vi "cargarDatoEstadistica.vi"(11 "IndiceAUltimoValor\nAgregadoEnLaTabla":i32=1) -> ()   [LabVIEW 2014]
uses:
  claseEstadistica/claseEstadistica.lvclass
panel:
  out "dataReading":T1
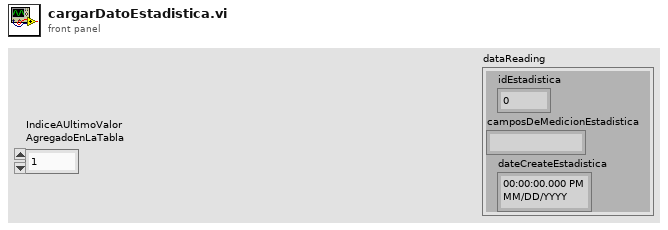
[diagram p1: front panel]
types:
  T1 = cluster{"idEstadistica":dbl, "camposDeMedicionEstadistica":string, "dateCreateEstadistica":timestamp}
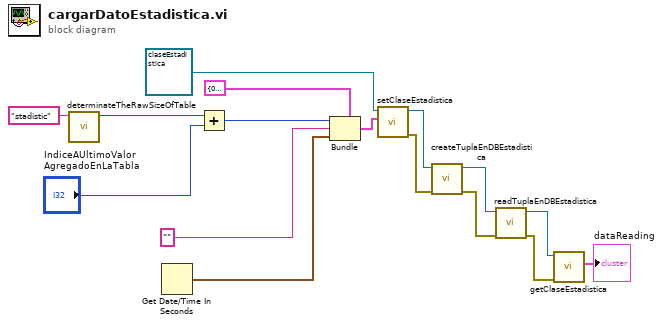
[diagram p0: block diagram]
diagram:
  n1 = call "determinateTheRawSizeOfTable.vi"("tableName"="stadistic") -> ("sizeOfTableInNumberRaw"=w3:i32)  [unwired: 8 in, 1 out]
  n2 = Get Date/Time In Seconds() -> (seconds since 1Jan1904=w14:timestamp)
  n3 = Add(x=w3, y="IndiceAUltimoValor\nAgregadoEnLaTabla") -> (x+y=w15:i32)
  n4 = Bundle(cluster=T1 {"idEstadistica"=0.0, "camposDeMedicionEstadistica"="", "dateCreateEstadistica"=timestamp(0 s since 1904-01-01)} ("dataToSet"), "idEstadistica"=w15, "camposDeMedicionEstadistica"="", "dateCreateEstadistica"=w14) -> (w10:T1)
  n5 = call "setClaseEstadistica.vi"("dataToSet"=w10, "claseEstadistica in"=refnum<class "claseEstadistica.lvclass"> refnum ("claseEstadistica.lvclass")) -> ("error out"=w8:errorcluster, "claseEstadistica out"=w9:refnum<class "claseEstadistica.lvclass">)  [unwired: 8 in]
  n6 = call "createTuplaEnDBEstadistica.vi"("error in"=w8, "claseEstadistica in"=w9) -> ("error out"=w6:errorcluster, "claseEstadistica out"=w7:refnum<class "claseEstadistica.lvclass">)  [unwired: 8 in]
  n7 = call "readTuplaEnDBEstadistica.vi"("error in"=w6, "claseEstadistica in"=w7) -> ("error out"=w4:errorcluster, "claseEstadistica out"=w5:refnum<class "claseEstadistica.lvclass">)  [unwired: 8 in]
  n8 = call "getClaseEstadistica.vi"("claseEstadistica in"=w5, "error in"=w4) -> ("dataReading"=→"dataReading":T1)  [unwired: 6 in, 2 out]
